vi "scanTest.vi"() -> ()   [LabVIEW 2012]
uses:
  <userlib>/atmcd32d.llb/ReadMode_mode typedef.ctl
  <userlib>/atmcd32d.llb/AcquisitionMode_mode typedef.ctl
  <userlib>/atmcd32d.llb/TriggerMode_mode typedef.ctl
  <userlib>/atmcd32d.llb/Spool_method typedef.ctl
panel:
  in  "Path":path
  in  "File Name":string
  in  "START SCAN":bool
  in  "Startup cmd":string
  in  "Frame":dbl
  in  "Delay":dbl
  in  "synch cmd":string
  in  "cycle cmd":string
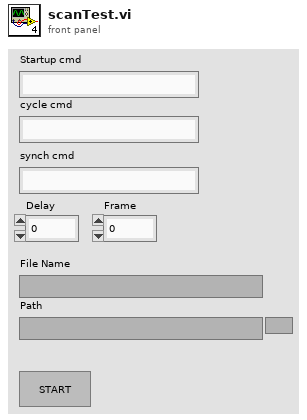
[diagram p1: front panel]
types:
  T1 = typedef "ReadMode_mode typedef.ctl" = enum16{"Full Vertical Binning", "Multi-Track", "Random-Track", "Single-Track", "Image"}
  T2 = typedef "AcquisitionMode_mode typedef.ctl" = enum16{"Reserved (0)", "Single Scan", "Accumulate", "Kinetics", "Fast Kinetics", "Run Till Abort", "Reserved (6)", "Reserved (7)", "Reserved (8)", "Time Delayed Integration"}
  T3 = typedef "TriggerMode_mode typedef.ctl" = enum16{"Internal", "External", "N/A (2)", "N/A (3)", "N/A (4)", "N/A (5)", "External Start", "External Exposure (Bulb)", "N/A (8)", "External FVB EM", "Software", "N/A (11)", "External Charge Shifting"}
  T4 = typedef "Spool_method typedef.ctl" = enum16{"32-bit", "Depends", "16-bit", "Multiple Directory", "Spool to RAM disk", "16-bit FITS", "SIF", "16-buit TIFF", "Multiple Directory Compressed"}
  T5 = cluster{"DeviceID":string, "Channel":string, "param1":dbl, "Operation":string}
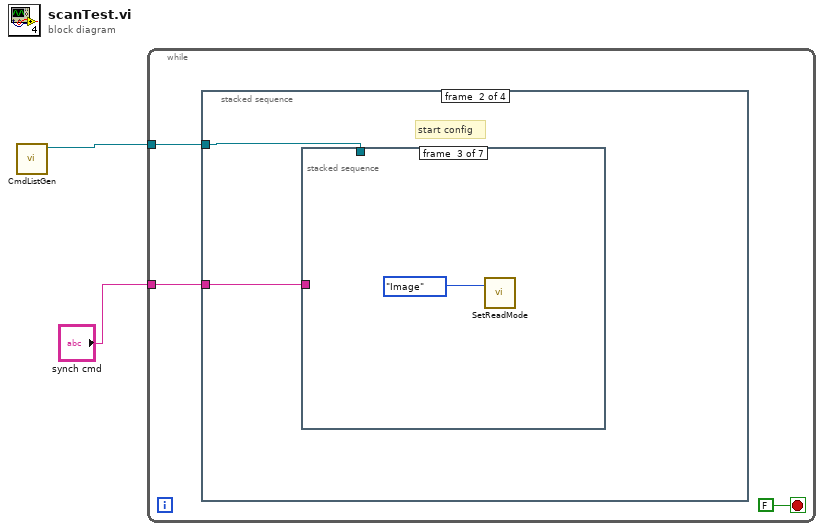
[diagram p0: block diagram]
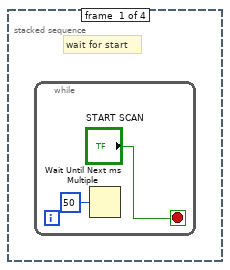
[diagram p2: hidden frame]
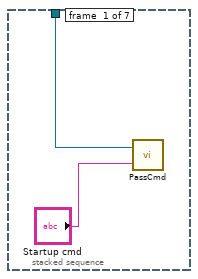
[diagram p3: hidden frame]
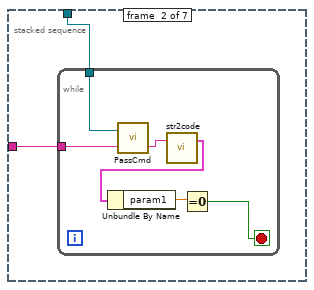
[diagram p4: hidden frame]
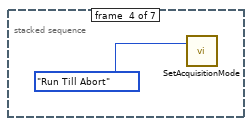
[diagram p5: hidden frame]
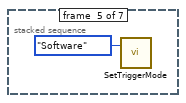
[diagram p6: hidden frame]
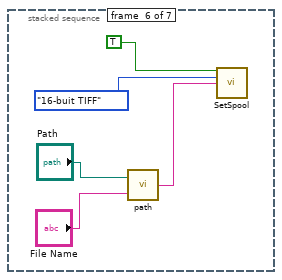
[diagram p7: hidden frame]
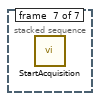
[diagram p8: hidden frame]
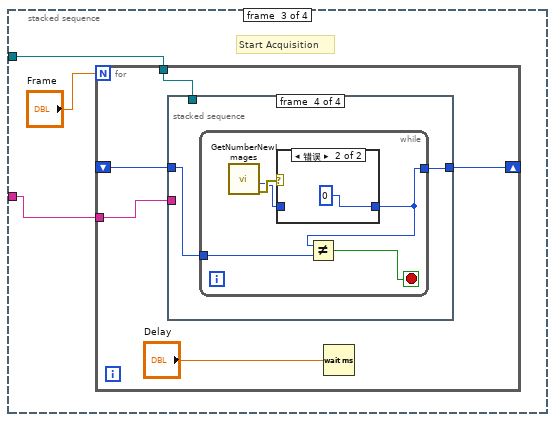
[diagram p9: hidden frame]
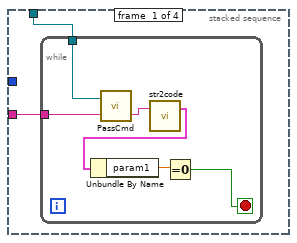
[diagram p10: hidden frame]
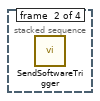
[diagram p11: hidden frame]
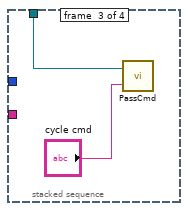
[diagram p12: hidden frame]
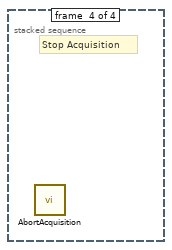
[diagram p14: hidden frame]
diagram:
  n1 = call "CmdListGen.vi"() -> ("MsgList"=w2:refnum<queue>)  [unwired: 1 in, 3 out]
  n2 = while {
    tunnel: w2 -> [w4]
    tunnel: "synch cmd" -> [w3]
    stop <- FALSE stop-if-true
    n3 = stacked-sequence {
      tunnel: w4 -> [_ w9 w29 _]
      tunnel: w3 -> [_ w8 w28 _]
      frame #0 {
        # "wait for start"
        n4 = while {
          stop <- "START SCAN" stop-if-true
          n5 = Wait Until Next ms Multiple(millisecond multiple=u32 50 ("毫秒倍数")) -> ()  [unwired: 1 out]
        }
      }
      frame #1 {
        # "start config"
        n6 = stacked-sequence {
          tunnel: w9 -> [w11 w13 _ _ _ _ _]
          tunnel: w8 -> [_ w12 _ _ _ _ _]
          frame #0 {
            n7 = call "PassCmd.vi"("cmd in"="Startup cmd", "list ref"=w11) -> ()  [unwired: 2 out]
          }
          frame #1 {
            n8 = while {
              tunnel: w13 -> [w19]
              tunnel: w12 -> [w18]
              stop <- w14 stop-if-true
              n9 = call "PassCmd.vi"("cmd in"=w18, "list ref"=w19) -> ("str out"=w17:string)  [unwired: 1 out]
              n10 = call "str2code.vi"("input"=w17) -> ("Output"=w16:T5)  [unwired: 1 in, 1 out]
              n11 = Unbundle By Name(w16) -> ("param1"=w15:dbl)
              n12 = Equal To 0?(x=w15) -> (x = 0?=w14:bool)
            }
          }
          frame #2 {
            n13 = call <userlib>:"SetReadMode.vi"("mode"=ReadMode_mode_typedef."Image") -> ()  [unwired: 1 in, 2 out]
          }
          frame #3 {
            n14 = call <userlib>:"SetAcquisitionMode.vi"("mode"=AcquisitionMode_mode_typedef."Run Till Abort") -> ()  [unwired: 1 in, 2 out]
          }
          frame #4 {
            n15 = call <userlib>:"SetTriggerMode.vi"("mode"=TriggerMode_mode_typedef."Software") -> ()  [unwired: 1 in, 2 out]
          }
          frame #5 {
            n16 = call "path.vi"("file"="File Name", "path_in"="Path") -> ("path_out"=w23:string)
            n17 = call <userlib>:"SetSpool.vi"("active"=TRUE, "method"=Spool_method_typedef."16-buit TIFF", "name"=w23) -> ()  [unwired: 11 in, 2 out]
          }
          frame #6 {
            n18 = call <userlib>:"StartAcquisition.vi"() -> ()  [unwired: 2 in, 2 out]
          }
        }
      }
      frame #2 {
        # "Start Acquisition"
        n19 = for {
          N: "Frame" -> [_]
          tunnel: w29 -> [w35]
          tunnel: w28 -> [w34]
          shift-right: [w31] -> _
          shift-left: _ -> [w32]
          n20 = stacked-sequence {
            tunnel: w35 -> [w36 _ w45 _]
            tunnel: w34 -> [w37 _ _ _]
            tunnel: w32 -> [_ _ _ w46]
            tunnel: [_ _ _ w47] -> w31
            frame #0 {
              n21 = while {
                tunnel: w36 -> [w43]
                tunnel: w37 -> [w42]
                stop <- w38 stop-if-true
                n22 = call "PassCmd.vi"("cmd in"=w42, "list ref"=w43) -> ("str out"=w41:string)  [unwired: 1 out]
                n23 = call "str2code.vi"("input"=w41) -> ("Output"=w40:T5)  [unwired: 1 in, 1 out]
                n24 = Unbundle By Name(w40) -> ("param1"=w39:dbl)
                n25 = Equal To 0?(x=w39) -> (x = 0?=w38:bool)
              }
            }
            frame #1 {
              n26 = call <userlib>:"SendSoftwareTrigger.vi"() -> ()  [unwired: 1 in, 2 out]
            }
            frame #2 {
              n27 = call "PassCmd.vi"("cmd in"="cycle cmd", "list ref"=w45) -> ()  [unwired: 2 out]
            }
            frame #3 {
              n28 = while {
                tunnel: w46 -> [w52]
                tunnel: [w48] -> w47
                stop <- w51 stop-if-true
                n29 = call <userlib>:"GetNumberNewImages.vi"() -> ("error out"=w50:errorcluster, "last"=w49:i32)  [unwired: 4 in, 2 out]
                n30 = case shown="错误" w50 {
                  tunnel: w49 -> [w53 _]
                  tunnel: [w53 0] -> w48
                  frame No Error {
                  }
                  frame Error {
                  }
                }
                n31 = Not Equal?(x=w48, y=w52) -> (x != y?=w51:bool)
              }
            }
          }
          n32 = Wait (ms)(milliseconds to wait="Delay") -> ()  [unwired: 1 out]
        }
      }
      frame #3 {
        # "Stop Acquisition"
        n33 = call <userlib>:"AbortAcquisition.vi"() -> ()  [unwired: 2 in, 2 out]
      }
    }
  }
